vi "Wczytanie_ustawien_AI_DI.vi"(8 "error in (no error)":errorcluster, 9 "Kanały cyfrowe in":refnum<vi>, 10 "AI referencje Array":refnum<vi>[](array[refnum]), 11 "configuration file path":path) -> (0 "error out":errorcluster, 1 "output cluster":T4, 2 "Analog konfig":T1[](array[typedef]) {"Numer" min=1 max=8 step=1})   [LabVIEW 2014]
doc: "Wczytuje ustawienia kanałów analogowych i cyfrowych\nz jednego wspólnego pliku INI"
uses:
  Kontrolki/GUI/DI_aktywacja.ctl
  Kontrolki/GUI/AI_parametry.ctl
  Kontrolki/GUI/AI_typ pom.ctl
  Kontrolki/GUI/AI_wartosc.ctl
  <vilib>/Utility/config.llb/Read Key (String).vi
  <vilib>/Utility/config.llb/NI_LVConfig.lvlib
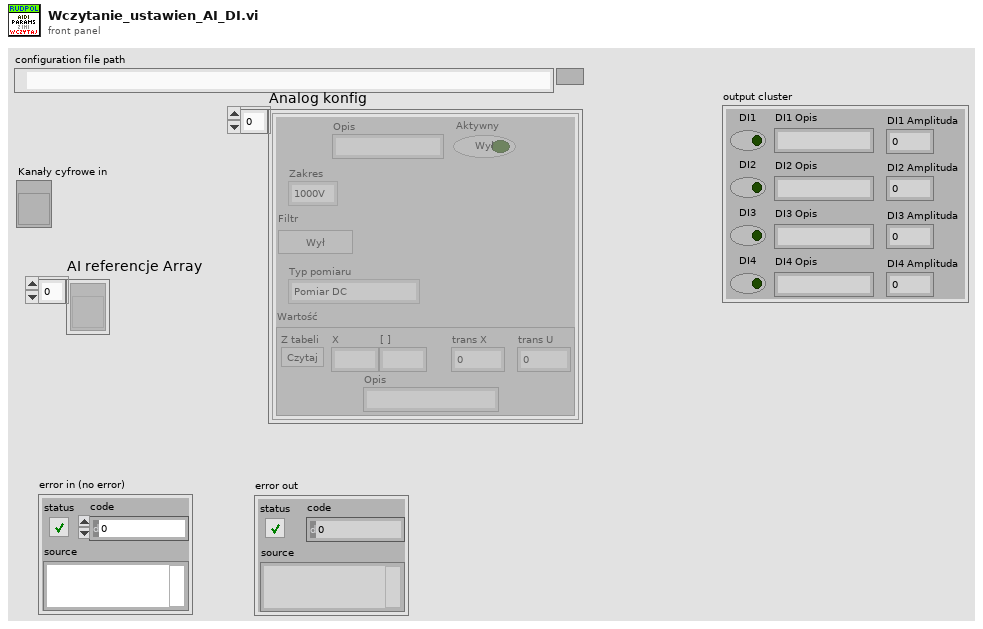
[diagram p1: front panel]
types:
  T1 = typedef "AI_parametry.ctl" = cluster{"Numer":u8, "Opis":string, "Zakres":enum16{"1000V", "300V", "30V", "3V", "0,3V"}, "Filtr":bool, "Typ pomiaru":T2, "Aktywny":bool, "Wartość":T3}
  T2 = typedef "AI_typ pom.ctl" = enum16{"Pomiar DC", "Pomiar AC+DC", "Pomiar AC"}
  T3 = typedef "AI_wartosc.ctl" = cluster{"X":string, "[ ]":string, "trans X":dbl, "trans U":dbl, "Z tabeli":bool, "Opis":string}
  T4 = typedef "DI_aktywacja.ctl" = cluster{"DI1":bool, "DI2":bool, "DI3":bool, "DI4":bool, "DI1 Opis":string, "DI2 Opis":string, "DI3 Opis":string, "DI4 Opis":string, "DI1 Amplituda":dbl, "DI2 Amplituda":dbl, "DI3 Amplituda":dbl, "DI4 Amplituda":dbl}
  T5 = typedef "NI_LVConfig.lvlib/Config Data RefNum.ctl" = refnum<k1>
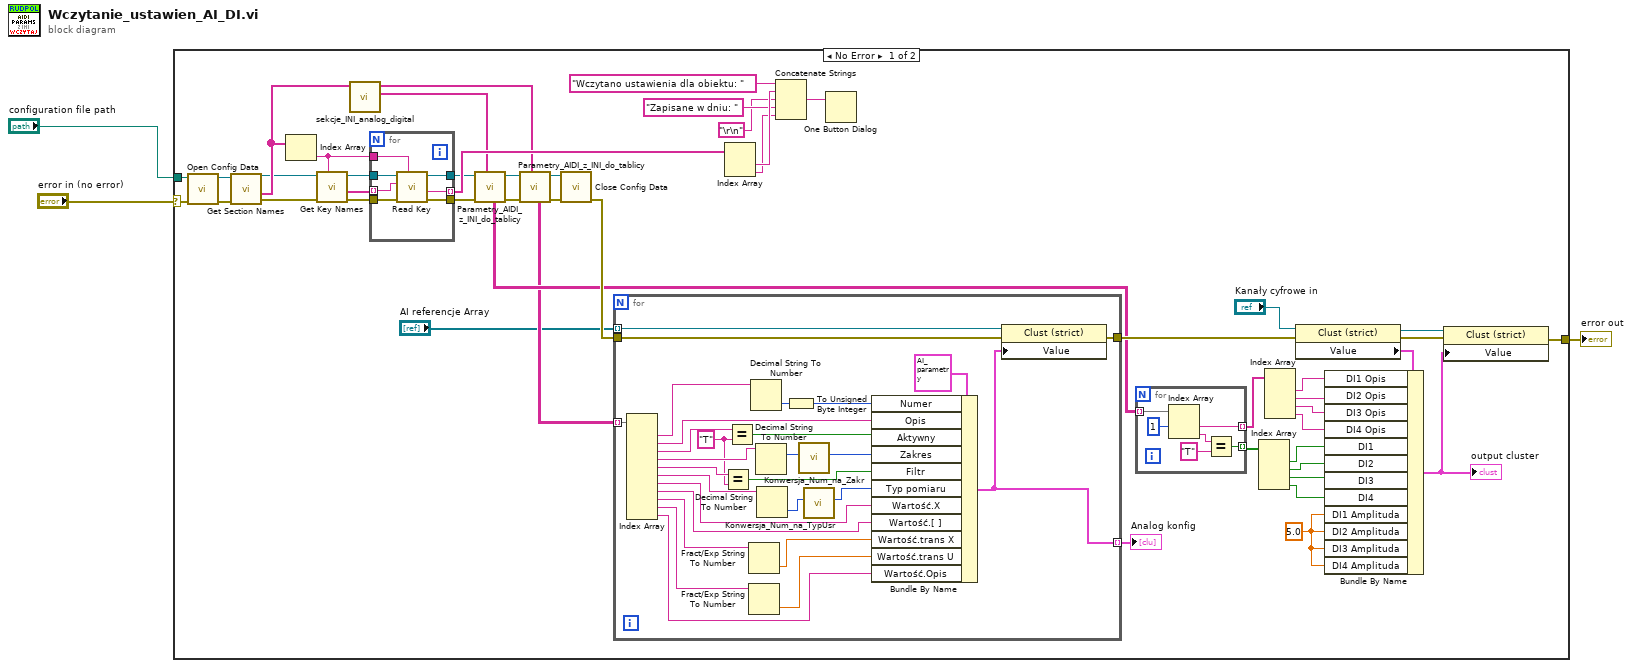
[diagram p0: block diagram]
diagram:
  n1 = case shown="No Error" "error in (no error)" {
    selector: "error in (no error)" -> [w6 w94]
    tunnel: "configuration file path" -> [w50 _]
    tunnel: [w7 w94] -> w2
    frame No Error {
      w17 = 5.0 ("DI1 Amplituda")
      n2 = call <vilib>:"Open Config Data.vi"("error in (no error)"=w6, "configuration file path"=w50) -> ("error out"=w52:errorcluster, "refnum"=w51:T5)  [unwired: 7 in, 1 out]
      n3 = call <vilib>:"Get Section Names.vi"("error in (no error)"=w52, "refnum"=w51) -> ("error out"=w47:errorcluster, "section names"=w49:string[], "refnum out"=w48:T5)  [unwired: 7 in]
      n4 = Index Array(array=w49) -> (element=w44:string)  [unwired: 1 in]
      n5 = call <vilib>:"Get Key Names.vi"("section"=w44, "error in (no error)"=w47, "refnum"=w48) -> ("error out"=w46:errorcluster, "key names"=w43:string[], "refnum out"=w45:T5)  [unwired: 5 in, 1 out]
      n6 = call "sekcje_INI_analog_digital.vi"("section names"=w49) -> ("DI sections"=w16:string[], "AI sections"=w11:string[])  [unwired: 9 in]
      n7 = for {
        tunnel: w45 -> [w93]
        tunnel: w46 -> [w92]
        tunnel: [w91] -> w34
        tunnel: [w90] -> w35
        tunnel: w44 -> [w89]
        tunnel: w43 -> [w88] mode=indexing
        tunnel: [w87] -> w42 mode=indexing
        n8 = call-poly <vilib>:"Read Key.vi"("section"=w89, "error in (no error)"=w92, "key"=w88, "refnum"=w93) -> ("error out"=w91:errorcluster, "value"=w87:string, "refnum out"=w90:T5)  [unwired: 4 in, 1 out]
      }
      n9 = call "Parametry_AIDI_z_INI_do_tablicy.vi"("Sections in"=w16, "error in (no error)"=w34, "Refnum in"=w35) -> ("error out"=w12:errorcluster, "Refnum out"=w13:T5, "Keys out"=w15:string[][])  [unwired: 6 in]
      n10 = call "Parametry_AIDI_z_INI_do_tablicy.vi"("Sections in"=w11, "error in (no error)"=w12, "Refnum in"=w13) -> ("error out"=w8:errorcluster, "Refnum out"=w9:T5, "Keys out"=w10:string[][])  [unwired: 6 in]
      n11 = call <vilib>:"Close Config Data.vi"("error in (no error)"=w8, "refnum"=w9) -> ("error out"=w33:errorcluster)  [unwired: 8 in, 1 out]
      n12 = for {
        tunnel: w10 -> [w86] mode=indexing
        tunnel: "AI referencje Array" -> [w60] mode=indexing
        tunnel: w33 -> [w64]
        tunnel: [w63] -> w28
        tunnel: [w59] -> w4 mode=indexing
        w74 = "T" ("y")
        n13 = Index Array(array=w86) -> (element #1=w85:string, element #2=w82:string, element #3=w80:string, element #4=w78:string, element #5=w76:string, element #6=w73:string, element #7=w71:string, element #8=w70:string, element #9=w69:string, element #10=w67:string, element #11=w65:string)  [unwired: 11 in]
        n14 = Equal?(x=w76, y=w74) -> (x = y?=w75:bool)
        n15 = Equal?(x=w80, y=w74) -> (x = y?=w79:bool)
        n16 = Fract/Exp String To Number(string=w69) -> (number=w68:dbl)  [unwired: 3 in, 1 out]
        n17 = Fract/Exp String To Number(string=w67) -> (number=w66:dbl)  [unwired: 3 in, 1 out]
        n18 = Decimal String To Number(string=w85) -> (number=w84:i32)  [unwired: 2 in, 1 out]
        n19 = Decimal String To Number(string=w78) -> (number=w81:i32)  [unwired: 2 in, 1 out]
        n20 = Decimal String To Number(string=w73) -> (number=w72:i32)  [unwired: 2 in, 1 out]
        n21 = To Unsigned Byte Integer(number=w84) -> (unsigned 8bit integer=w83:u8)
        n22 = call "Konwersja_Num_na_Zakr.vi"("Zakres No"=w81) -> ("Zakres out"=w77:enum16{"1000V", "300V", "30V", "3V", "0,3V"})  [unwired: 10 in]
        n23 = call "Konwersja_Num_na_TypUsr.vi"("Zakres No"=w72) -> ("Typ pomiaru"=w62:T2)  [unwired: 10 in]
        n24 = Bundle By Name(cluster=T1 {"Numer"=1, "Opis"="Kanał 1", "Zakres"=enum."1000V", "Filtr"=FALSE, "Typ pomiaru"=enum."Pomiar DC", "Aktywny"=FALSE, "Wartość"={"X"="U", "[ ]"="V", "trans X"=1.0, "trans U"=1.0, "Z tabeli"=FALSE, "Opis"=""}} ("AI_parametry"), "Numer"=w83, "Opis"=w82, "Aktywny"=w79, "Zakres"=w77, "Filtr"=w75, "Typ pomiaru"=w62, "Wartość.X"=w71, "Wartość.[ ]"=w70, "Wartość.trans X"=w68, "Wartość.trans U"=w66, "Wartość.Opis"=w65) -> (w59:T1)
        n25 = property class="Clust (strict)"(reference=w60, error in=w64, "Value"=w59) -> (error out=w63:errorcluster)  [unwired: 1 out]
      }
      "Analog konfig" <- w4
      n26 = Index Array(array=w42) -> (element #1=w40:string, element #2=w38:string)  [unwired: 2 in]
      n27 = Concatenate Strings("Wczytano ustawienia dla obiektu: " ("string"), w40, "\r\n", "Zapisane w dniu: " ("string"), w38) -> (w36:string)
      n28 = One Button Dialog(message=w36) -> ()  [unwired: 1 in, 1 out]
      n29 = for {
        tunnel: w15 -> [w58] mode=indexing
        tunnel: [w57] -> w27 mode=indexing
        tunnel: [w53] -> w22 mode=indexing
        n30 = Index Array(array=w58, index #1=1 ("index")) -> (element #1=w57:string, element #2=w55:string)  [unwired: 1 in]
        n31 = Equal?(x=w55, y="T") -> (x = y?=w53:bool)
      }
      n32 = Index Array(array=w22) -> (element #1=w21:bool, element #2=w20:bool, element #3=w19:bool, element #4=w18:bool)  [unwired: 4 in]
      n33 = Index Array(array=w27) -> (element #1=w26:string, element #2=w25:string, element #3=w24:string, element #4=w23:string)  [unwired: 4 in]
      n34 = property class="Clust (strict)"(reference="Kanały cyfrowe in", error in=w28) -> (reference out=w14:refnum<vi>, error out=w30:errorcluster, "Value"=w31:T4)
      n35 = Bundle By Name(cluster=w31, "DI1 Opis"=w26, "DI2 Opis"=w25, "DI3 Opis"=w24, "DI4 Opis"=w23, "DI1"=w21, "DI2"=w20, "DI3"=w19, "DI4"=w18, "DI1 Amplituda"=w17, "DI2 Amplituda"=w17, "DI3 Amplituda"=w17, "DI4 Amplituda"=w17) -> (w32:T4)
      "output cluster" <- w32
      n36 = property class="Clust (strict)"(reference=w14, error in=w30, "Value"=w32) -> (error out=w7:errorcluster)  [unwired: 1 out]
    }
    frame Error {
    }
  }
  "error out" <- w2
